vi "Configure Current Stirrer.vi"(8 "error in (no error)":errorcluster, 10 "Stirrer Option":i32=1 min=1 max=3 step=1, 11 "heater_explorer in":refnum<class "heater_explorer.lvclass">) -> (0 "error out":errorcluster, 3 "heater_explorer out":refnum<class "heater_explorer.lvclass">)   [LabVIEW 2020, in "polar_bear_plus_drivers.lvlib" / "heater_explorer.lvclass"]
doc: "Configures the current stirrer to one of 1 = magnetic (internal, default), 2 = Overhead (small), 3 = Overhead (large) or Tumble Stirrer."
uses:
  <instrlib>/RxnRover/Driver Polar Bear Plus/heater_explorer/heater_explorer.lvclass
  <instrlib>/RxnRover/Driver Polar Bear Plus/heater_explorer/heater_explorer.lvclass/heater_explorer.ctl
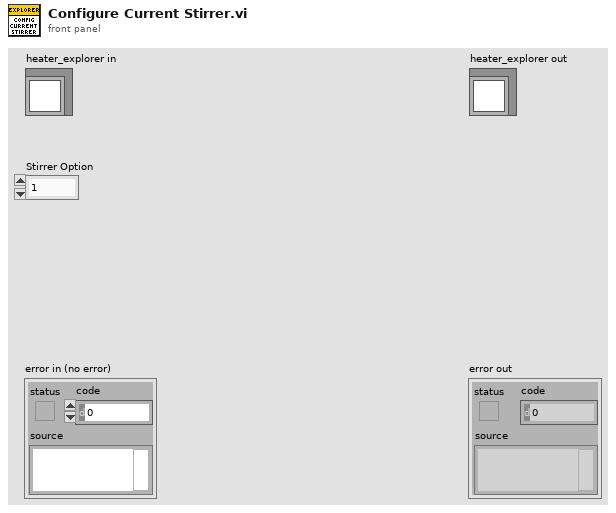
[diagram p1: front panel]
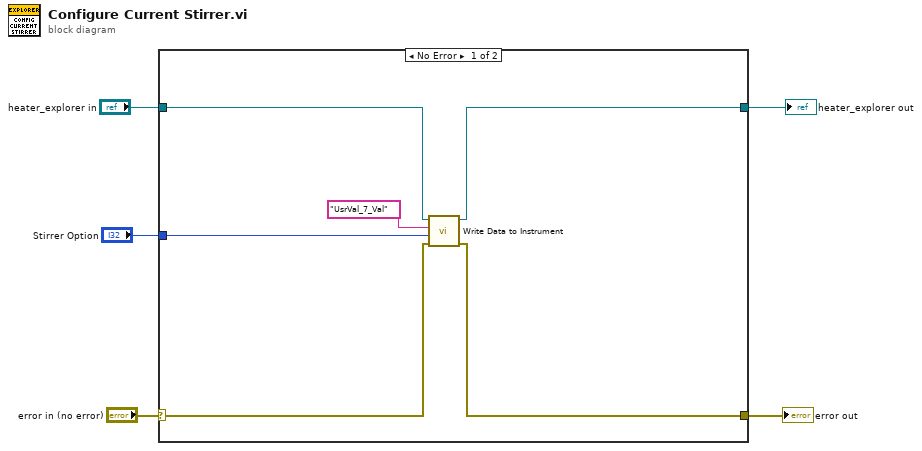
[diagram p0: block diagram]
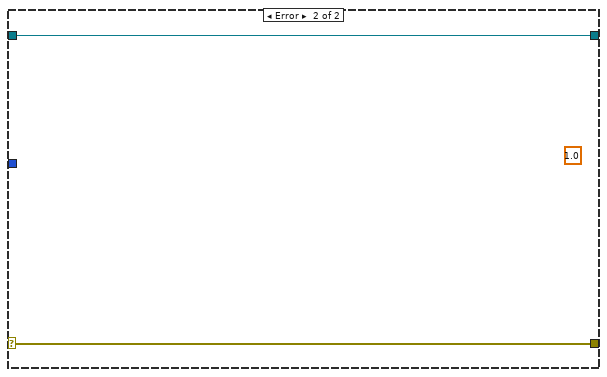
[diagram p2: hidden frame]
diagram:
  n1 = case shown="No Error" "error in (no error)" {
    selector: "error in (no error)" -> [w11 w12]
    tunnel: [w10 w12] -> w4
    tunnel: "heater_explorer in" -> [w8 w13]
    tunnel: [w7 w13] -> w2
    tunnel: "Stirrer Option" -> [w6 _]
    frame No Error {
      n2 = call-dynamic "Write Data to Instrument.vi"("error in (no error)"=w11, "Value to Send"=w6, "Address"="UsrVal_7_Val", "heater_parent in"=w8) -> ("error out"=w10:errorcluster, "heater_parent out"=w7:refnum<class "heater_explorer.lvclass">)  [unwired: 6 in]
    }
    frame Error {
      (unwired) 1.0 ("Value Read")
    }
  }
  "error out" <- w4
  "heater_explorer out" <- w2
